vi "Elevation Calibration.vi"(4 "Abort":refnum<vi>, 6 "Dialog Indicator":refnum<vi>, 7 "Angles":refnum<vi>, 8 "error in":errorcluster, 9 "Step [um]":dbl=100.0, 10 "#steps":i32=10, 11 "Manipulator Interface":T2) -> (0 "error out":errorcluster)   [LabVIEW 2012, in "Targeting Unit.lvlib"]
uses:
  Targeting Unit.lvlib
  <vilib>/Analysis/Matrix/Datatypes/RealMatrix.ctl
  <vilib>/Analysis/baseanly.llb/Unimode.vi
  <vilib>/Analysis/NI_AALBase.lvlib
  <vilib>/Analysis/Matrix/NI_Matrix.lvlib
panel:
  out "Histogram Graph":T1(graph)
  out "Elevation":dbl
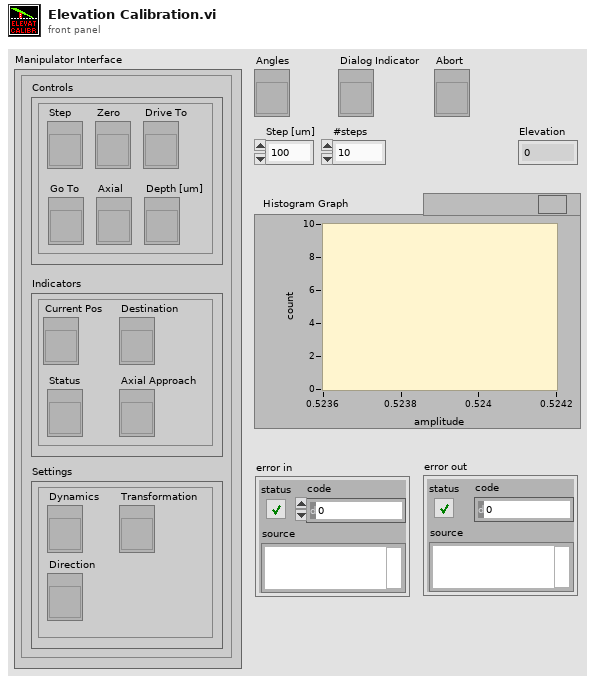
[diagram p1: front panel]
types:
  T1 = cluster{"X Values":dbl[], "Histogram: h(x)":i32[]}
  T2 = cluster{"Indicators":cluster{"Current Pos":refnum<vi>, "Destination":refnum<vi>, "Status":refnum<vi>, "Axial Approach":refnum<vi>}, "Settings":cluster{"Dynamics":refnum<vi>, "Transformation":refnum<vi>, "Direction":refnum<vi>}, "Controls":cluster{"Zero":refnum<vi>, "Step":refnum<vi>, "Drive To":refnum<vi>, "Go To":refnum<vi>, "Axial":refnum<vi>, "Depth [um]":refnum<vi>}}
  T3 = cluster{"Step length [um]":dbl, "Interstep Interval [ms]":u32, "Initial Speed [um/s]":dbl, "Max Speed [um/s]":dbl, "Acceleration [um/s^2]":dbl, "Max Depth [um]":dbl, "Max Penetration [um]":dbl}
  T4 = cluster{"X [um]":dbl, "Y [um]":dbl, "Z [um]":dbl}
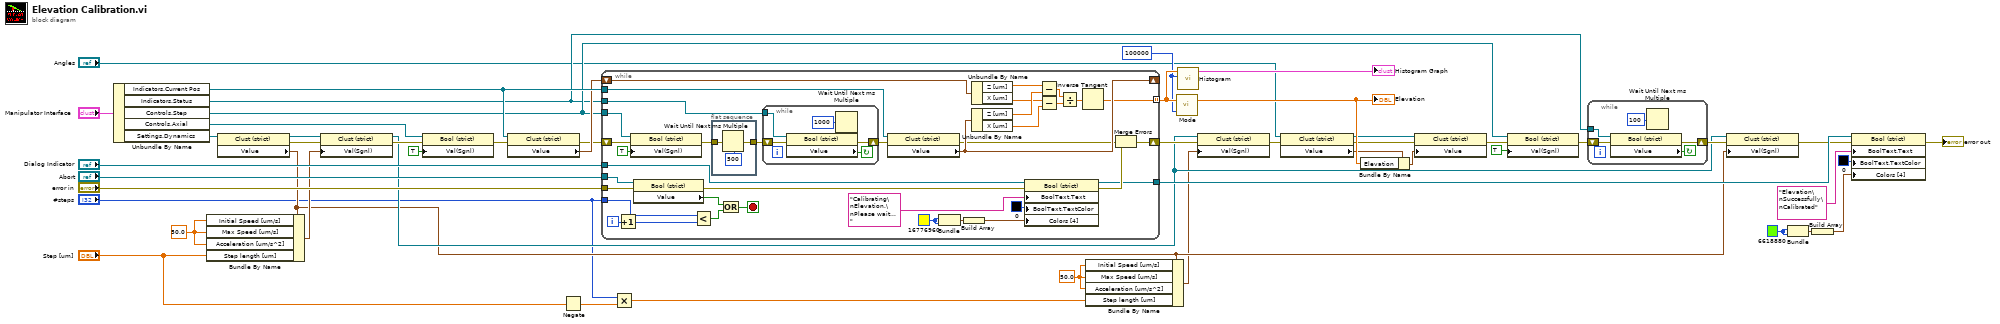
[diagram p0: block diagram]
diagram:
  w7 = 100000 ("intervals")
  w12 = u32 6618880
  w19 = 50.0 ("Initial Speed [um/s]")
  w29 = 50.0 ("Initial Speed [um/s]")
  n1 = Unbundle By Name("Manipulator Interface") -> ("Indicators.Current Pos"=w47:refnum<vi>, "Indicators.Status"=w40:refnum<vi>, "Controls.Step"=w43:refnum<vi>, "Controls.Axial"=w33:refnum<vi>, "Settings.Dynamics"=w31:refnum<vi>)
  n2 = property class="Clust (strict)"(reference=w31) -> (reference out=w28:refnum<vi>, error out=w26:errorcluster, "Value"=w20:T3)  [unwired: 1 in]
  n3 = Bundle By Name(cluster=w20, "Initial Speed [um/s]"=w29, "Max Speed [um/s]"=w29, "Acceleration [um/s^2]"=w29, "Step length [um]"="Step [um]") -> (w30:T3)
  n4 = property class="Clust (strict)"(reference=w28, error in=w26, "Val(Sgnl)"=w30) -> (reference out=w21:refnum<vi>, error out=w27:errorcluster)
  n5 = property class="Bool (strict)"(reference=w33, error in=w27, "Val(Sgnl)"=TRUE) -> (error out=w48:errorcluster)  [unwired: 1 out]
  n6 = property class="Clust (strict)"(reference=w47, error in=w48) -> (error out=w32:errorcluster, "Value"=w46:T4)  [unwired: 1 out]
  n7 = Negate(x="Step [um]") -> (-x=w15:dbl)
  n8 = while {
    tunnel: w43 -> [w86]
    tunnel: w40 -> [w85]
    tunnel: w47 -> [w84]
    shift-right: [w75] -> _
    shift-left: w46 -> [w78]
    tunnel: [w74] -> w10 mode=indexing
    tunnel: "Abort" -> [w73]
    tunnel: "#steps" -> [w55]
    shift-right: [w64] -> w25
    shift-left: w32 -> [w56]
    tunnel: "error in" -> [w69]
    tunnel: "Dialog Indicator" -> [w61]
    tunnel: [w60] -> w36
    i -> [w70]
    stop <- w71 stop-if-true
    w51 = u32 16776960
    n9 = Increment(x=w70) -> (x+1=w54:i32)
    n10 = property class="Bool (strict)"(reference=w86, error in=w56, "Val(Sgnl)"=TRUE ("Value (Signaling)")) -> (error out=w57:errorcluster)  [unwired: 1 out]
    n11 = property class="Bool (strict)"(reference=w73, error in=w69) -> (error out=w66:errorcluster, "Value"=w72:bool)  [unwired: 1 out]
    n12 = Less?(x=w55, y=w54) -> (x < y?=w53:bool)
    n13 = flat-sequence {
      tunnel: [w88] -> w58
      tunnel: w57 -> [w88]
      frame #0 {
        n14 = Wait Until Next ms Multiple(millisecond multiple=u32 500) -> ()  [unwired: 1 out]
      }
    }
    n15 = Or(x=w72, y=w53) -> (x .or. y?=w71:bool)
    n16 = while {
      tunnel: w85 -> [w89]
      shift-right: [w90] -> w65
      shift-left: w58 -> [w91]
      stop <- w93 continue-if-true
      n17 = property class="Bool (strict)"(reference=w89, error in=w91) -> (error out=w90:errorcluster, "Value"=w93:bool)  [unwired: 1 out]
      n18 = Wait Until Next ms Multiple(millisecond multiple=u32 1000) -> ()  [unwired: 1 out]
    }
    n19 = property class="Clust (strict)"(reference=w84, error in=w65) -> (error out=w63:errorcluster, "Value"=w75:T4)  [unwired: 1 out]
    n20 = Bundle(w51, w51) -> (w52:cluster{u32, u32})  [unwired: 1 in]
    n21 = Build Array(w52) -> (w50:cluster{u32, u32}[])
    n22 = Unbundle By Name(w78) -> ("Z [um]"=w77:dbl, "X [um]"=w76:dbl)
    n23 = Unbundle By Name(w75) -> ("Z [um]"=w83:dbl, "X [um]"=w82:dbl)
    n24 = property class="Bool (strict)"(reference=w61, error in=w66, "BoolText.Text"="Calibrating\nElevation.\nPlease wait..." ("Window Title (\"\")"), "BoolText.TextColor"=u32 0, "Colors [4]"=w50) -> (reference out=w60:refnum<vi>, error out=w62:errorcluster)
    n25 = Subtract(x=w77, y=w83) -> (x-y=w81:dbl)
    n26 = Subtract(x=w76, y=w82) -> (x-y=w80:dbl)
    n27 = Divide(x=w81, y=w80) -> (x/y=w79:dbl)
    n28 = Inverse Tangent(1:w79) -> (0:w74:dbl)
    n29 = Merge Errors(w63, w62) -> (w64:errorcluster)
  }
  n30 = Multiply(x="#steps", y=w15) -> (x*y=w14:dbl)
  n31 = Bundle By Name(cluster=w20, "Initial Speed [um/s]"=w19, "Max Speed [um/s]"=w19, "Acceleration [um/s^2]"=w19, "Step length [um]"=w14) -> (w17:T3)
  n32 = call-poly <vilib>:"Mode.vi"("intervals"=w7, "X"=w10) -> ("mode"=w8:dbl)  [unwired: 1 out]
  "Elevation" <- w8
  n33 = call <vilib>:"Histogram.vi"("intervals"=w7, "X"=w10) -> ("Histogram Graph"=→"Histogram Graph":T1)  [unwired: 6 in, 3 out]
  n34 = property class="Clust (strict)"(reference=w21, error in=w25, "Val(Sgnl)"=w17) -> (error out=w5:errorcluster)  [unwired: 1 out]
  n35 = property class="Clust (strict)"(reference="Angles", error in=w5) -> (reference out=w1:refnum<vi>, error out=w6:errorcluster, "Value"=w4:cluster{"Azimut":dbl, "Elevation":dbl})
  n36 = Bundle By Name(cluster=w4, "Elevation"=w8) -> (w3:cluster{"Azimut":dbl, "Elevation":dbl})
  n37 = property class="Clust (strict)"(reference=w1, error in=w6, "Value"=w3) -> (error out=w24:errorcluster)  [unwired: 1 out]
  n38 = property class="Bool (strict)"(reference=w43, error in=w24, "Val(Sgnl)"=TRUE ("Value (Signaling)")) -> (error out=w41:errorcluster)  [unwired: 1 out]
  n39 = while {
    tunnel: w40 -> [w94]
    shift-right: [w95] -> w23
    shift-left: w41 -> [w96]
    stop <- w98 continue-if-true
    n40 = property class="Bool (strict)"(reference=w94, error in=w96) -> (error out=w95:errorcluster, "Value"=w98:bool)  [unwired: 1 out]
    n41 = Wait Until Next ms Multiple(millisecond multiple=u32 100) -> ()  [unwired: 1 out]
  }
  n42 = property class="Clust (strict)"(reference=w21, error in=w23, "Val(Sgnl)"=w20) -> (error out=w22:errorcluster)  [unwired: 1 out]
  n43 = Bundle(w12, w12) -> (w13:cluster{u32, u32})  [unwired: 1 in]
  n44 = Build Array(w13) -> (w11:cluster{u32, u32}[])
  n45 = property class="Bool (strict)"(reference=w36, error in=w22, "BoolText.Text"="Elevation\nSuccessfully\nCalibrated" ("Window Title (\"\")"), "BoolText.TextColor"=u32 0, "Colors [4]"=w11) -> (error out=→"error out":errorcluster)  [unwired: 1 out]
